vi "Compression Iter.vi"(7 "i":i32, 10 "Var In":u32[](array[numeric]) format="0x%08x", 11 "w[i]":u32 format="0x%08x") -> (2 "Var":u32[](array[numeric]) format="0x%08x")   [LabVIEW 2018, in "Crypto.lvlib" / "SHA-256.lvclass"]
uses:
  SHA-256.lvclass
  Sigma1.vi
  Choice.vi
  K.vi
  Sigma0.vi
  Major.vi
panel:
  # "a"
  # "b"
  # "c"
  # "d"
  # "e"
  # "f"
  # "g"
  # "h"
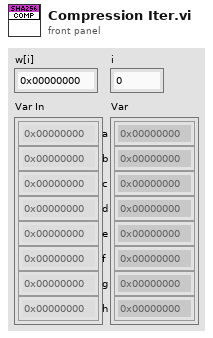
[diagram p1: front panel]
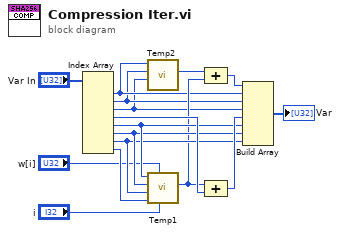
[diagram p0: block diagram]
diagram:
  n1 = Index Array(array="Var In") -> (element #1=w4:u32, element #2=w3:u32, element #3=w2:u32, element #4=w14:u32, element #5=w11:u32, element #6=w10:u32, element #7=w9:u32, element #8=w8:u32)  [unwired: 8 in]
  n2 = call "Temp2.vi"("c"=w2, "b"=w3, "a"=w4) -> ("Temp 2"=w1:u32)  [unwired: 8 in]
  n3 = call "Temp1.vi"("i"="i", "w[i]"="w[i]", "h"=w8, "g"=w9, "f"=w10, "e"=w11) -> ("Temp 1"=w7:u32)  [unwired: 5 in]
  n4 = Compound Arithmetic op=ADD(w1, w7) -> (w16:u32)
  n5 = Compound Arithmetic op=ADD(w7, w14) -> (w15:u32)
  n6 = Build Array(w16, w4, w3, w2, w15, w11, w10, w9) -> (→"Var":u32[])
